vi "labview-embedded-main.vi"() -> ()   [LabVIEW 2014]
uses:
  SubVI/Websockets/Controls/TCP State Machine States.ctl
  Globals/applicaiton-globals.vi
  SubVI/Websockets/Globals/messages.vi
panel:
  out "Error Out":errorcluster
  in  "Error In":errorcluster
  out "New Message":string
  out "New Command":string
  out "Devices":i32
  out "TCP State Machine States":T1
  out "Running":bool
  in  "Stop":bool
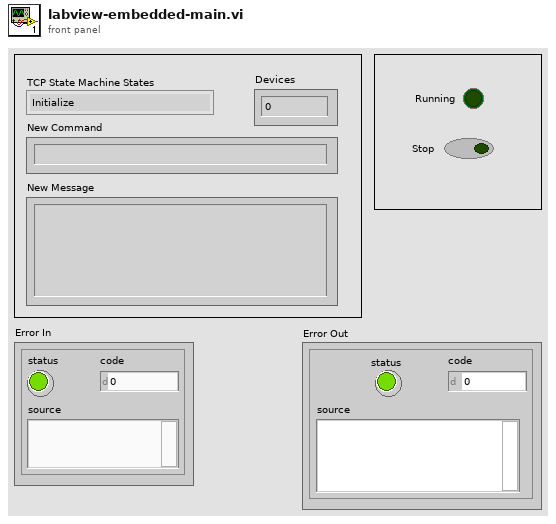
[diagram p1: front panel]
types:
  T1 = typedef "TCP State Machine States.ctl" = enum16{"Initialize", "Status Check", "Read Data", "Stop"}
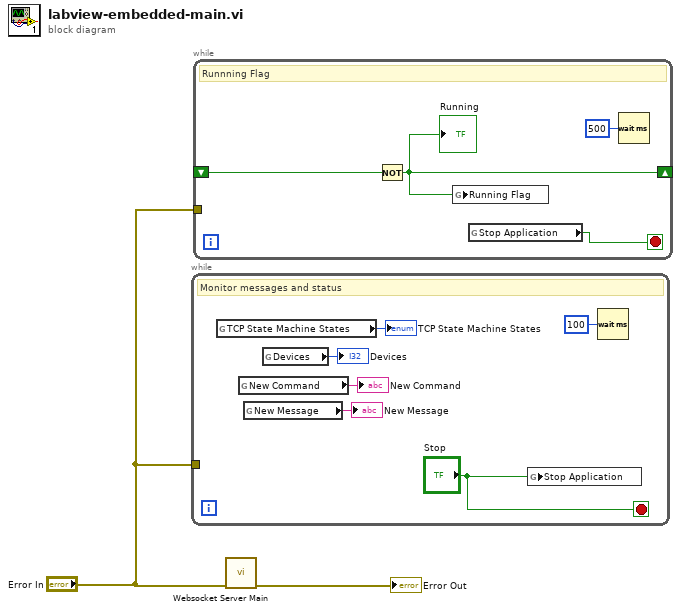
[diagram p0: block diagram]
diagram:
  n1 = while {
    tunnel: "Error In" -> [_]
    stop <- "Stop" stop-if-true
    # "Monitor messages and status"
    n2 = global read "messages.vi" "TCP State Machine States"() -> (→"TCP State Machine States":T1)
    n3 = global read "messages.vi" "New Command"() -> (→"New Command":string)
    n4 = global read "messages.vi" "New Message"() -> (→"New Message":string)
    n5 = global read "messages.vi" "Devices"() -> (→"Devices":i32)
    n6 = global write "applicaiton-globals.vi" "Stop Application"("Stop") -> ()
    n7 = Wait (ms)(milliseconds to wait=u32 100) -> ()  [unwired: 1 out]
  }
  n8 = while {
    shift-right: [w10] -> _
    shift-left: _ -> [w9]
    tunnel: "Error In" -> [_]
    stop <- w11 stop-if-true
    # "Runnning Flag"
    n9 = Not(x=w9) -> (.not. x?=w10:bool)
    "Running" <- w10
    n10 = global write "applicaiton-globals.vi" "Running Flag"(w10) -> ()
    n11 = global read "applicaiton-globals.vi" "Stop Application"() -> (w11:bool)
    n12 = Wait (ms)(milliseconds to wait=u32 500) -> ()  [unwired: 1 out]
  }
  n13 = call "Websocket Server Main.vi"("Error In"="Error In") -> ("Error Out"=→"Error Out":errorcluster)  [unwired: 10 in]
